vi "Obtain Request Events.vi"(8 "error in (no error)":errorcluster, 10 "Create New?":bool) -> (0 "error out":errorcluster, 2 "Thermal Chamber Controller_DQMH Request Events":T1)   [LabVIEW 2015, in "Thermal Chamber Controller_DQMH.lvlib"]
doc: "This VI Obtains/Creates the Requests events that will be used for other modules to communicate with the module that owns this VI. These Requests events will be accessed only via Public API methods for this module.\n\n<b>NOTE</b>: The contents of this VI are automatically generated and modified by the <b>Tools > Delacor > DQMH</b> utilities. Consider using those utilities instead of making your own modifications to this VI.\n_____\nBased on Delacor QMH Project Template 2.0.0.62.\n____\nDelacor QMH Thermal Chamber Examples 4.0.0.21\nCopyright (c) 2018, Delacor"
uses:
  Thermal Chamber Controller_DQMH.lvlib
  Request Events--cluster.ctl
  Stop Argument--cluster.ctl
  Show Panel Argument--cluster.ctl
  Hide Panel Argument--cluster.ctl
  Get Module Execution Status Argument--cluster.ctl
  Show Diagram Argument--cluster.ctl
  Update Set Point Argument--cluster.ctl
  Update Ramp Rate Argument--cluster.ctl
  Update Heater State Argument--cluster.ctl
  Heater State--enum.ctl
  Update Chamber Status Argument--cluster.ctl
  Request and Wait for Status Argument--cluster.ctl
  Request and Wait for Status (Reply Payload)--cluster.ctl
panel:
  # "NOTE: The contents of this VI are automatically generated and modified by the Tools > Delacor > DQMH utilities. Consider using those utilities instead of making your own modifications to this VI."
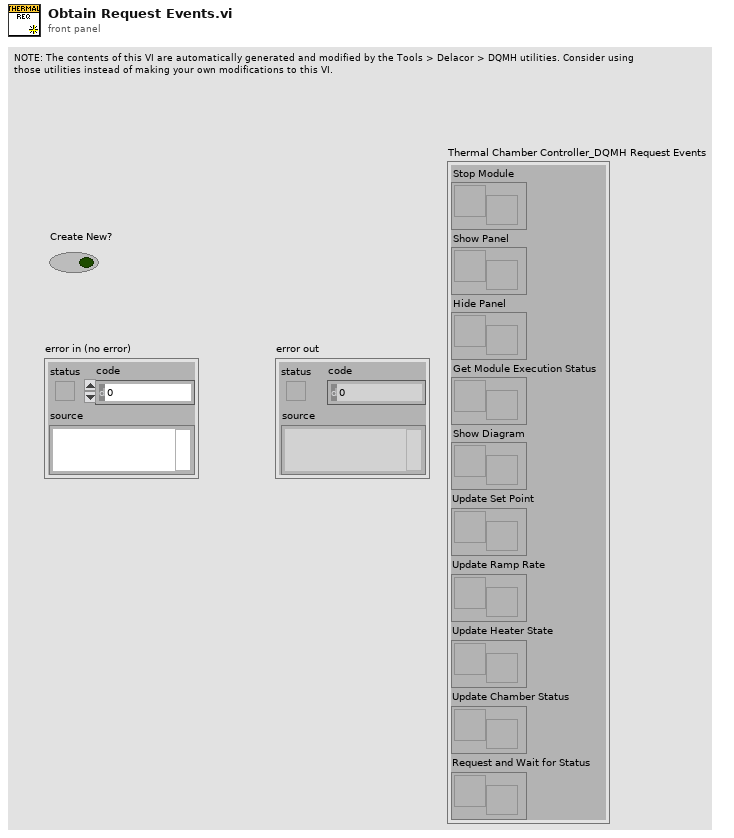
[diagram p1: front panel]
types:
  T1 = typedef "Thermal Chamber Controller_DQMH.lvlib/Request Events--cluster.ctl" = cluster{"Stop Module":refnum<user-event>, "Show Panel":refnum<user-event>, "Hide Panel":refnum<user-event>, "Get Module Execution Status":refnum<user-event>, "Show Diagram":refnum<user-event>, "Update Set Point":refnum<user-event>, "Update Ramp Rate":refnum<user-event>, "Update Heater State":refnum<user-event>, "Update Chamber Status":refnum<user-event>, "Request and Wait for Status":refnum<user-event>}
  T2 = typedef "Thermal Chamber Controller_DQMH.lvlib/Hide Panel Argument--cluster.ctl" = cluster{"Hide Panel?":bool}
  T3 = typedef "Thermal Chamber Controller_DQMH.lvlib/Show Panel Argument--cluster.ctl" = cluster{"Show Panel?":bool}
  T4 = typedef "Thermal Chamber Controller_DQMH.lvlib/Request and Wait for Status Argument--cluster.ctl" = cluster{"Wait Notifier":refnum<notifier>}
  T5 = typedef "Thermal Chamber Controller_DQMH.lvlib/Update Chamber Status Argument--cluster.ctl" = cluster{"Temperature Set Point":dbl, "Temperature Ramp Rate":dbl, "Heater State":T6, "Actual Temperature":dbl}
  T6 = typedef "Thermal Chamber Controller_DQMH.lvlib/Heater State--enum.ctl" = enum16{"Heater Enabled", "Heater Disabled"}
  T7 = typedef "Thermal Chamber Controller_DQMH.lvlib/Update Heater State Argument--cluster.ctl" = cluster{"Heater State":T6}
  T8 = typedef "Thermal Chamber Controller_DQMH.lvlib/Update Ramp Rate Argument--cluster.ctl" = cluster{"Temperature Ramp Rate":dbl}
  T9 = typedef "Thermal Chamber Controller_DQMH.lvlib/Update Set Point Argument--cluster.ctl" = cluster{"Temperature Set Point":dbl}
  T10 = typedef "Thermal Chamber Controller_DQMH.lvlib/Show Diagram Argument--cluster.ctl" = cluster{"Debug?":bool}
  T11 = typedef "Thermal Chamber Controller_DQMH.lvlib/Get Module Execution Status Argument--cluster.ctl" = cluster{"Running?":bool}
  T12 = typedef "Thermal Chamber Controller_DQMH.lvlib/Stop Argument--cluster.ctl" = cluster{"Origin":string, "Exit via Stop Module Req?":bool, "Wait for Module to stop?":bool}
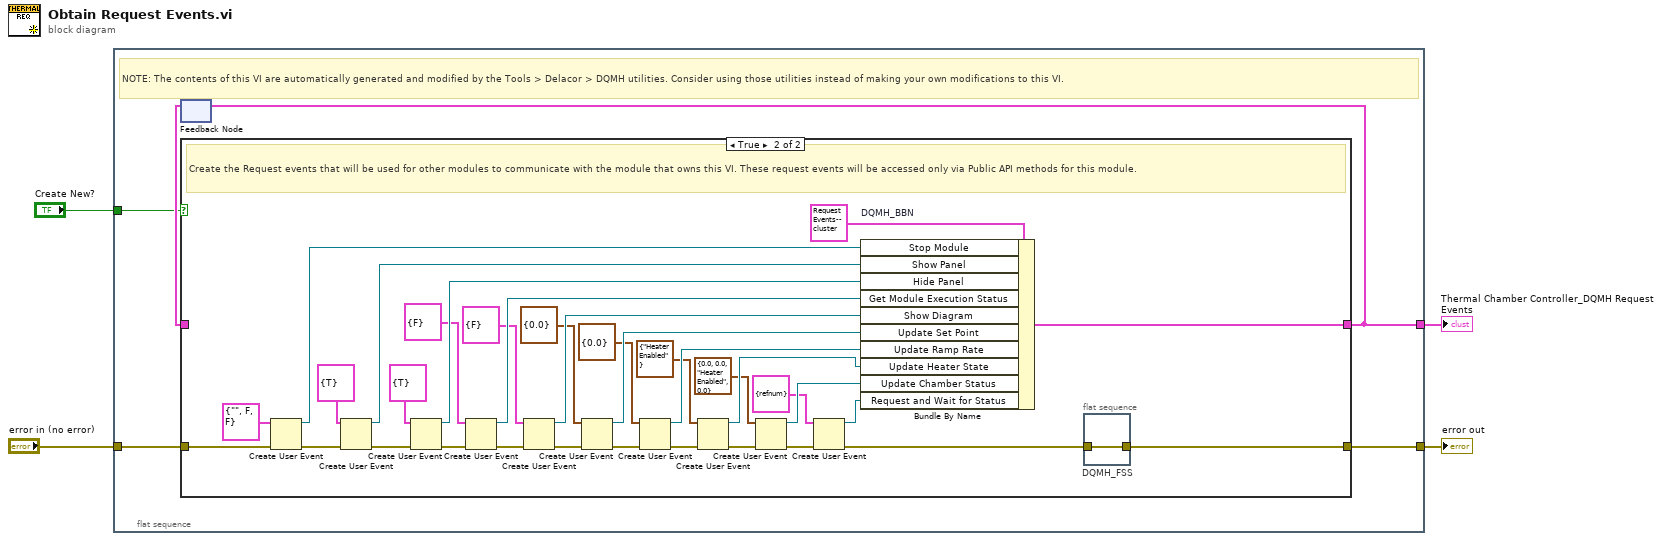
[diagram p0: block diagram]
diagram:
  n1 = flat-sequence {
    tunnel: [w9] -> w4
    tunnel: "error in (no error)" -> [w8]
    tunnel: [w6] -> w2
    tunnel: "Create New?" -> [w5]
    frame #0 {
      # "NOTE: The contents of this VI are automatically generated and modified by the Tools > Delacor > DQMH utilities. Consider using those utilities instead of making your own modifications to this VI."
      n2 = feedback #1() -> (w7:T1)  [unwired: 1 in]
      n3 = case shown="True" w5 {
        tunnel: [w10 w35] -> w9
        tunnel: w8 -> [w10 w45]
        tunnel: [w11 w42] -> w6
        tunnel: w7 -> [w11 _]
        frame False {
          # "Obtain the Request events that were created in a previous call to this VI."
        }
        frame True {
          # "Create the Request events that will be used for other modules to communicate with the module that owns this VI. These request events will be accessed only via Public API methods for this module."
          n4 = Create User Event(user event datatype=T12 {"Origin"="", "Exit via Stop Module Req?"=FALSE, "Wait for Module to stop?"=FALSE} ("Stop Argument"), error in=w45) -> (user event=w43:refnum<user-event>, error out=w40:errorcluster)
          n5 = Create User Event(user event datatype=T3 {"Show Panel?"=TRUE} ("Show Panel Argument"), error in=w40) -> (user event=w39:refnum<user-event>, error out=w38:errorcluster)
          n6 = Create User Event(user event datatype=T2 {"Hide Panel?"=TRUE} ("Hide Panel Argument"), error in=w38) -> (user event=w37:refnum<user-event>, error out=w36:errorcluster)
          n7 = Create User Event(user event datatype=T11 {"Running?"=FALSE} ("Get Module Execution Status Argument"), error in=w36) -> (user event=w33:refnum<user-event>, error out=w34:errorcluster)
          n8 = Create User Event(user event datatype=T10 {"Debug?"=FALSE} ("Show Diagram Argument"), error in=w34) -> (user event=w30:refnum<user-event>, error out=w31:errorcluster)
          n9 = Create User Event(user event datatype=T9 {"Temperature Set Point"=0.0} ("Update Set Point Argument"), error in=w31) -> (user event=w27:refnum<user-event>, error out=w28:errorcluster)
          n10 = Create User Event(user event datatype=T8 {"Temperature Ramp Rate"=0.0} ("Update Ramp Rate Argument"), error in=w28) -> (user event=w24:refnum<user-event>, error out=w25:errorcluster)
          n11 = Create User Event(user event datatype=T7 {"Heater State"=enum."Heater Enabled"} ("Update Heater State Argument"), error in=w25) -> (user event=w21:refnum<user-event>, error out=w22:errorcluster)
          n12 = Create User Event(user event datatype=T5 {"Temperature Set Point"=0.0, "Temperature Ramp Rate"=0.0, "Heater State"=enum."Heater Enabled", "Actual Temperature"=0.0} ("Update Chamber Status Argument"), error in=w22) -> (user event=w18:refnum<user-event>, error out=w19:errorcluster)
          n13 = Create User Event(user event datatype=T4 {"Wait Notifier"=refnum} ("Request and Wait for Status Argument"), error in=w19) -> (user event=w15:refnum<user-event>, error out=w16:errorcluster)
          n14 = Bundle By Name "DQMH_BBN"(cluster=T1 {"Stop Module"=refnum, "Show Panel"=refnum, "Hide Panel"=refnum, "Get Module Execution Status"=refnum, "Show Diagram"=refnum, "Update Set Point"=refnum, "Update Ramp Rate"=refnum, "Update Heater State"=refnum, "Update Chamber Status"=refnum, "Request and Wait for Status"=refnum} ("output cluster"), "Stop Module"=w43, "Show Panel"=w39, "Hide Panel"=w37, "Get Module Execution Status"=w33, "Show Diagram"=w30, "Update Set Point"=w27, "Update Ramp Rate"=w24, "Update Heater State"=w21, "Update Chamber Status"=w18, "Request and Wait for Status"=w15) -> (w42:T1)
          n15 = flat-sequence "DQMH_FSS" {
            tunnel: w16 -> [w46]
            tunnel: [w46] -> w35
            frame #0 {
            }
          }
        }
      }
      n16 = feedback-in #1(w6) -> ()
    }
  }
  "Thermal Chamber Controller_DQMH Request Events" <- w2
  "error out" <- w4
